vi "Rx.vi"(8 "error in (no error)":errorcluster, 11 "Framework in":refnum<class "Framework.lvclass">) -> (0 "error out":errorcluster, 3 "Framework out":refnum<class "Framework.lvclass">)   [LabVIEW 2017, in "DSF Core.lvlib" / "Framework.lvclass"]
uses:
  Framework.lvclass
  Framework.lvclass/Framework.ctl
  Interfaces/Dispatcher/Command.ctl
  Scheduler/Scheduler.lvclass
  Interfaces/Dispatcher/Dispatcher Interface.lvclass
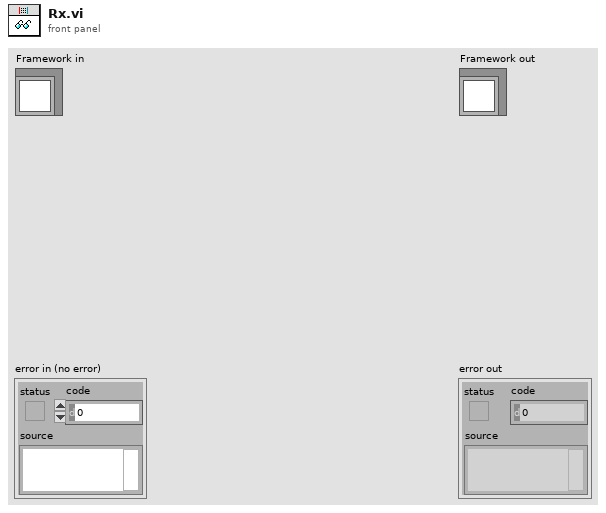
[diagram p1: front panel]
types:
  T1 = typedef "DSF Core.lvlib/Dispatcher Interface.lvclass/Command.ctl" = enum8{"Rx", "Tx", "Shutdown"}
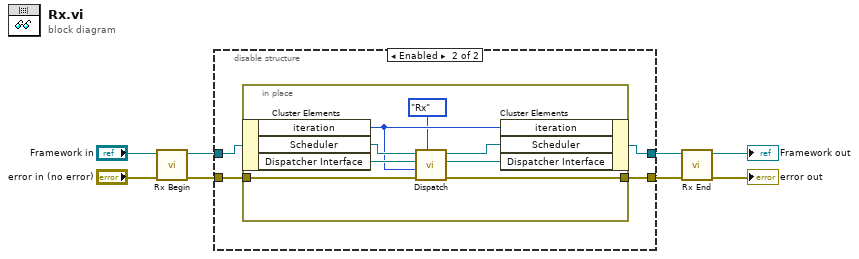
[diagram p0: block diagram]
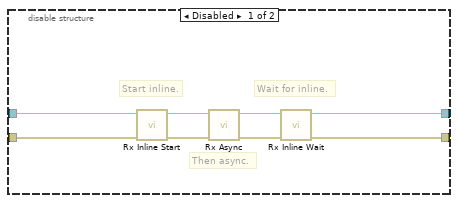
[diagram p2: hidden frame]
diagram:
  n1 = call "Rx Begin.vi"("error in (no error)"="error in (no error)", "Framework in"="Framework in") -> ("error out"=w6:errorcluster, "Framework out"=w1:refnum<class "Framework.lvclass">)  [unwired: 8 in]
  n2 = disable-structure shown="Enabled" {
    disable-tunnel: w1 -> [w16 w20]
    disable-tunnel: w6 -> [w15 w19]
    disable-tunnel: [w14 w18] -> w5
    disable-tunnel: [w13 w17] -> w4
    frame Disabled {
      # "Wait for inline."
      # "Start inline."
      # "Then async."
      n3 = call "Rx Inline Start.vi"("error in (no error)"=w15, "Framework in"=w16) -> ("error out"=w9:errorcluster, "Framework out"=w10:refnum<class "Framework.lvclass">)  [unwired: 8 in]
      n4 = call "Rx Async.vi"("error in (no error)"=w9, "Framework in"=w10) -> ("error out"=w12:errorcluster, "Framework out"=w11:refnum<class "Framework.lvclass">)  [unwired: 8 in]
      n5 = call "Rx Inline Wait.vi"("error in (no error)"=w12, "Framework in"=w11) -> ("error out"=w14:errorcluster, "Framework out"=w13:refnum<class "Framework.lvclass">)  [unwired: 8 in]
    }
    frame Enabled {
      n6 = in-place {
        in-place-border: w19 -> [w27]
        in-place-border: [w26] -> w18
        n7 = in-place-cluster #1(w20) -> ("iteration"=w22:u64, "Scheduler"=w28:refnum<class "Scheduler.lvclass">, "Dispatcher Interface"=w24:refnum<class "Dispatcher Interface.lvclass">)
        n8 = call "Dispatch.vi"("command"=Command."Rx", "error in (no error)"=w27, "framework iteration"=w22, "Dispatcher Interface in"=w24, "Scheduler in"=w28) -> ("error out"=w26:errorcluster, "Dispatcher Interface out"=w23:refnum<class "Dispatcher Interface.lvclass">, "Scheduler out"=w25:refnum<class "Scheduler.lvclass">)  [unwired: 4 in]
        n9 = in-place-cluster #1("iteration"=w22, "Scheduler"=w25, "Dispatcher Interface"=w23) -> (w17:refnum<class "Framework.lvclass">)
      }
    }
  }
  n10 = call "Rx End.vi"("error in (no error)"=w5, "Framework in"=w4) -> ("error out"=→"error out":errorcluster, "Framework out"=→"Framework out":refnum<class "Framework.lvclass">)  [unwired: 8 in]
